vi "Uncompact.vi"(11 "Compacted":string) -> (3 "Uncompacted":string)   [LabVIEW 2019, in "JSONtext.lvlib"]
uses:
  JSONtext.lvlib
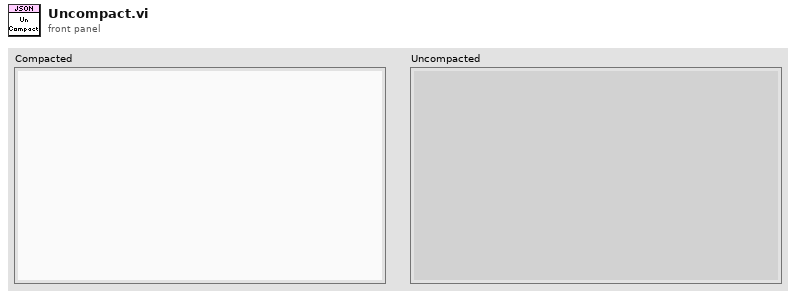
[diagram p1: front panel]
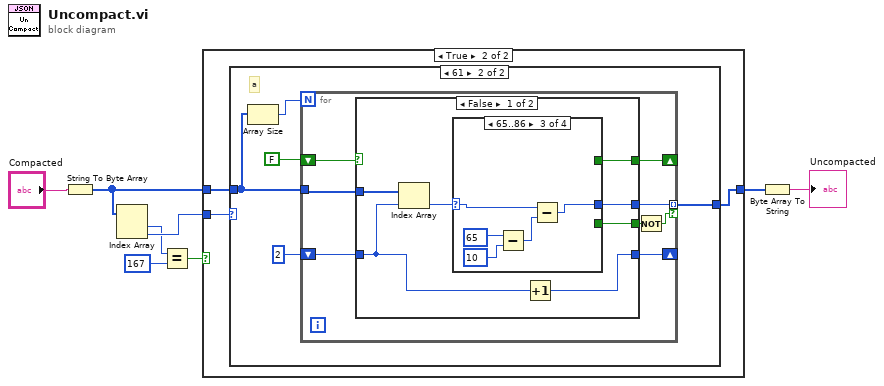
[diagram p0: block diagram]
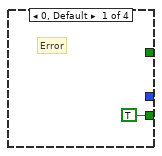
[diagram p4: hidden frame]
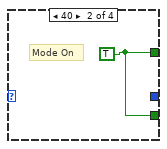
[diagram p5: hidden frame]
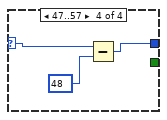
[diagram p6: hidden frame]
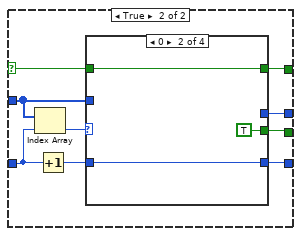
[diagram p7: hidden frame]
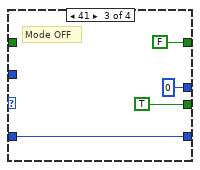
[diagram p9: hidden frame]
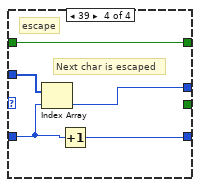
[diagram p10: hidden frame]
diagram:
  n1 = String To Byte Array(string="Compacted") -> (unsigned byte array=w5:u8[])
  n2 = Index Array(array=w5) -> (element #1=w2:u8, element #2=w6:u8)  [unwired: 2 in]
  n3 = Equal?(x=w2, y=u8 167) -> (x = y?=w4:bool)
  n4 = case shown="True" w4 {
    tunnel: w5 -> [w9 w12]
    tunnel: w6 -> [_ w11]
    tunnel: [w9 w10] -> w7
    frame False {
      # "Must be original format"
    }
    frame True {
      n5 = case shown="61" w11 {
        tunnel: w12 -> [w13 w14]
        tunnel: [w13 w16] -> w10
        frame 0, Default {
        }
        frame 97 {
          # "a"
          n6 = Array Size(array=w14) -> (size(s)=w15:i32)
          n7 = for {
            N: w15 -> [_]
            shift-right: [w22] -> _
            shift-left: FALSE -> [w26]
            shift-right: [w19] -> _
            shift-left: 2 -> [w24]
            tunnel: w14 -> [w25]
            tunnel: [w23] -> w16 mode=indexing if=w21
            n8 = case shown="False" w26 {
              selector: w26 -> [_ w48]
              tunnel: w25 -> [w33 w44]
              tunnel: w24 -> [w28 w47]
              tunnel: [w31 w51] -> w23
              tunnel: [w30 w49] -> w22
              tunnel: [w29 w50] -> w20
              tunnel: [w27 w45] -> w19
              frame False {
                n9 = Index Array(array=w33, index=w28) -> (element=w32:u8)
                n10 = case shown="65..86" w32 {
                  selector: w32 -> [_ _ w37 w43]
                  tunnel: [_ _ w36 w41] -> w31
                  tunnel: [_ w35 _ _] -> w30
                  tunnel: [TRUE w35 _ _] -> w29
                  frame 0, Default {
                    # "Error"
                  }
                  frame 40 {
                    w35 = TRUE
                    # "Mode On"
                  }
                  frame 65..86 {
                    n11 = Subtract(x=u8 65 ("y"), y=u8 10) -> (x-y=w38:u8)
                    n12 = Subtract(x=w37, y=w38) -> (x-y=w36:u8)
                  }
                  frame 47..57 {
                    n13 = Subtract(x=w43, y=u8 48) -> (x-y=w41:u8)
                  }
                }
                n14 = Increment(x=w28) -> (x+1=w27:i32)
              }
              frame True {
                n15 = Index Array(array=w44, index=w47) -> (element=w52:u8)
                n16 = Increment(x=w47) -> (x+1=w46:i32)
                n17 = case shown="0" w52 {
                  selector: w52 -> [w55 _ _ _]
                  tunnel: [w55 _ u8 0 w64] -> w51
                  tunnel: [_ TRUE TRUE _] -> w50
                  tunnel: [w54 w58 FALSE w63] -> w49
                  tunnel: w48 -> [w54 w58 _ w63]
                  tunnel: w46 -> [w53 w56 w59 w66]
                  tunnel: [w53 w56 w59 w65] -> w45
                  tunnel: w44 -> [_ _ _ w67]
                  frame Default {
                  }
                  frame 0 {
                  }
                  frame 41 {
                    # "Mode OFF"
                  }
                  frame 39 {
                    # "Next char is escaped"
                    # "escape"
                    n18 = Index Array(array=w67, index=w66) -> (element=w64:u8)
                    n19 = Increment(x=w66) -> (x+1=w65:i32)
                  }
                }
              }
            }
            n20 = Not(x=w20) -> (.not. x?=w21:bool)
          }
        }
      }
    }
  }
  n21 = Byte Array To String(unsigned byte array=w7) -> (string=→"Uncompacted":string)
